vi "openConnection_Publisher.vi"(8 "error in (no error)":errorcluster, 10 "TCP address":string="tcp://*:5555", 11 "LabVIEW-Python-Interface in":refnum<class "PyLVi.lvclass">) -> (0 "error out":errorcluster, 2 "connected":bool, 3 "LabVIEW-Python-Interface out":refnum<class "PyLVi.lvclass">)   [LabVIEW 2016, in "PyLVi.lvlib" / "PyLVi.lvclass"]
doc: "\"receive timeout\": timeout in ms. If value is negative, no timeout is set."
uses:
  PyLVi.lvclass
  <vilib>/addons/zeromq/socket_type.ctl
  PyLVi.lvclass/PyLVi.ctl
  <vilib>/addons/zeromq/zmq_context.lvclass
  <vilib>/addons/zeromq/zeromq.lvlib
  <vilib>/addons/zeromq/zmq_socket.lvclass
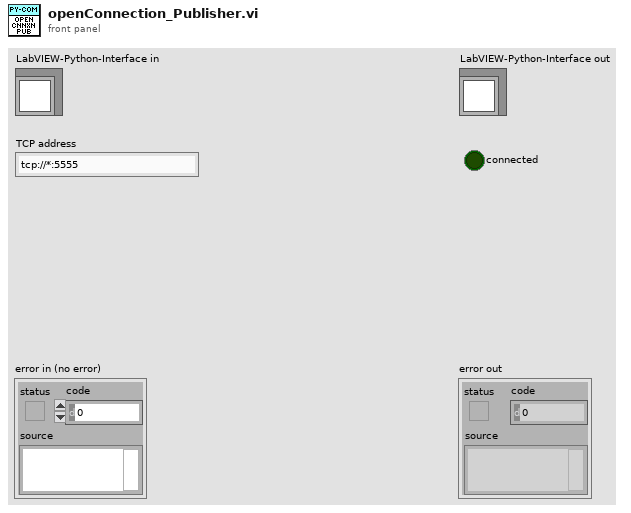
[diagram p1: front panel]
types:
  T1 = typedef "zeromq.lvlib/socket_type.ctl" = enum8{"ZMQ_PAIR", "ZMQ_PUB", "ZMQ_SUB", "ZMQ_REQ", "ZMQ_REP", "ZMQ_DEALER", "ZMQ_ROUTER", "ZMQ_PULL", "ZMQ_PUSH", "ZMQ_XPUB", "ZMQ_XSUB"}
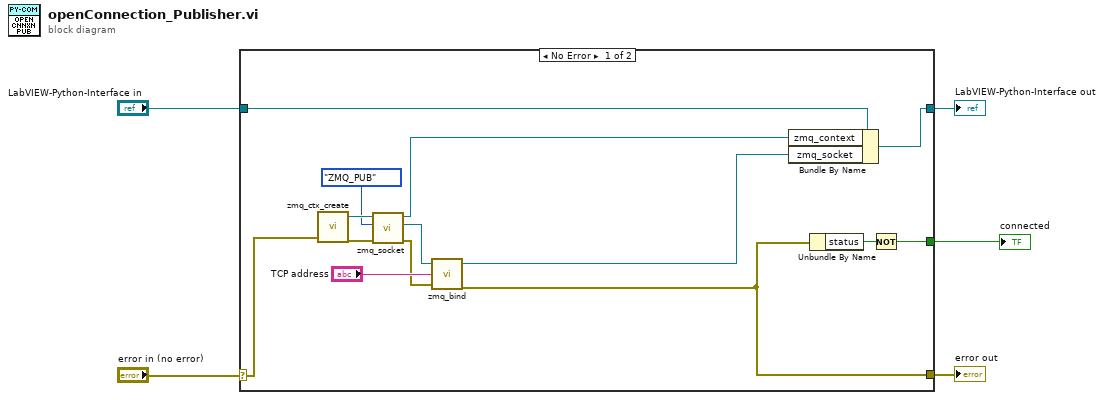
[diagram p0: block diagram]
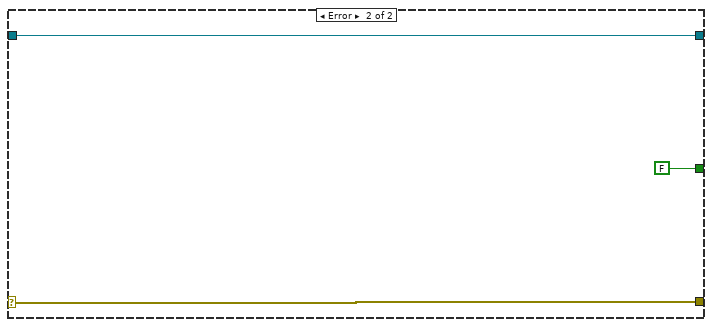
[diagram p2: hidden frame]
diagram:
  n1 = case shown="No Error" "error in (no error)" {
    selector: "error in (no error)" -> [w13 w22]
    tunnel: [w6 w22] -> w4
    tunnel: [w10 w21] -> w2
    tunnel: "LabVIEW-Python-Interface in" -> [w12 w21]
    tunnel: [w8 FALSE ("connected")] -> w1
    frame No Error {
      n2 = call <vilib>:"zmq_ctx_create.vi"("error in"=w13) -> ("error out"=w18:errorcluster, "context out"=w19:refnum<class "zmq_context.lvclass">)  [unwired: 3 in]
      n3 = call <vilib>:"zmq_socket.vi"("error in"=w18, "socket type"=socket_type."ZMQ_PUB", "context in"=w19) -> ("error out"=w14:errorcluster, "socket out"=w15:refnum<class "zmq_socket.lvclass">, "context out"=w11:refnum<class "zmq_context.lvclass">)  [unwired: 2 in]
      n4 = call <vilib>:"zmq_bind.vi"("error in"=w14, "endpoint"="TCP address", "socket in"=w15) -> ("error out"=w6:errorcluster, "socket out"=w7:refnum<class "zmq_socket.lvclass">)  [unwired: 1 in]
      n5 = Bundle By Name(cluster=w12, "zmq_context"=w11, "zmq_socket"=w7) -> (w10:refnum<class "PyLVi.lvclass">)
      n6 = Unbundle By Name(w6) -> ("status"=w9:bool)
      n7 = Not(x=w9) -> (.not. x?=w8:bool)
    }
    frame Error {
    }
  }
  "error out" <- w4
  "LabVIEW-Python-Interface out" <- w2
  "connected" <- w1
